vi "GetScriptItemName.vi"(8 "INI File Name":string, 9 "Class Name":string, 10 "Module Name":string, 11 "Script Name":string) -> (3 "Script Item Name":string, 5 "Action String":string)   [LabVIEW 2018]
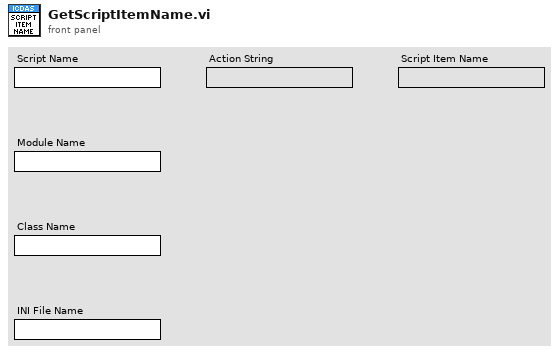
[diagram p1: front panel]
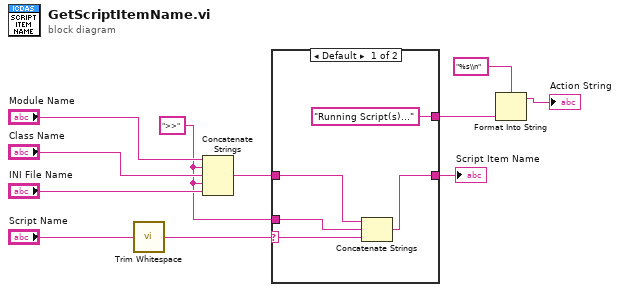
[diagram p0: block diagram]
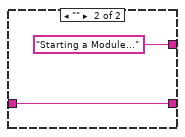
[diagram p2: hidden frame]
diagram:
  w6 = ">>" ("Module Name")
  n1 = call <vilib>:"Trim Whitespace.vi"("string"="Script Name") -> ("trimmed string"=w1:string)  [unwired: 1 in]
  n2 = Concatenate Strings("Module Name", w6, "Class Name", w6, "INI File Name") -> (w7:string)
  n3 = case shown="Default" w1 {
    selector: w1 -> [w16 _]
    tunnel: w7 -> [w12 w18]
    tunnel: w6 -> [w13 _]
    tunnel: [w15 w18] -> w5
    tunnel: ["Running Script(s)..." ("Module Name") "Starting a Module..." ("Module Name")] -> w2
    frame Default {
      n4 = Concatenate Strings(w12, w13, w16) -> (w15:string)
    }
    frame "" {
    }
  }
  "Script Item Name" <- w5
  n5 = Format Into String(format string="%s\\n", w2) -> (resulting string=→"Action String":string)  [unwired: 2 in, 1 out]
